vi "sendValue.vi"(8 "error in (no error)":errorcluster, 10 "data":variant, 11 "stopScan in":refnum<class "stopScan.lvclass">) -> (0 "error out":errorcluster, 2 "function return":i32, 3 "stopScan out":refnum<class "stopScan.lvclass">)   [LabVIEW 2016, in "SALLV_MtAtElectrometer_Messaging.lvlib" / "stopScan.lvclass"]
uses:
  stopScan.lvclass
  ts_sallv_MtAtElectrometer/DataTypes/command_stopScan.ctl
  ts_sallv_MtAtElectrometer/SALLV_MtAtElectrometer.lvlib
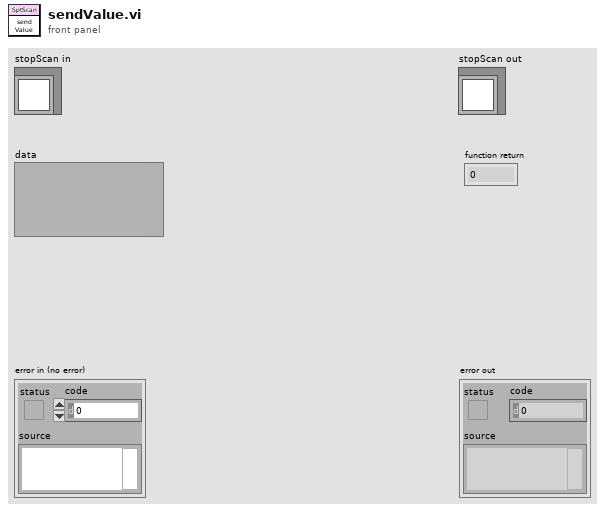
[diagram p1: front panel]
types:
  T1 = typedef "SALLV_MtAtElectrometer.lvlib/command_stopScan.ctl" = cluster{"value":bool}
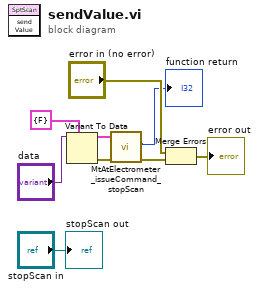
[diagram p0: block diagram]
diagram:
  n1 = Variant To Data(type=T1 {"value"=FALSE} ("command_stopScan_Ctl"), Variant="data") -> (data=w4:T1, error out=w5:errorcluster)  [unwired: 1 in]
  n2 = call "MtAtElectrometer_issueCommand_stopScan.vi"("error in (no error)"=w5, "command_stopScan_Ctl"=w4) -> ("error out"=w2:errorcluster, "function return"=→"function return":i32)  [unwired: 7 in, 1 out]
  n3 = Merge Errors("error in (no error)", w2) -> (→"error out":errorcluster)
  "stopScan out" <- "stopScan in"
